vi "FVT.vi"() -> ()   [LabVIEW 2024]
uses:
  <vilib>/Utility/file.llb/Write Delimited Spreadsheet (string).vi
panel:
  in  "CompRun":bool
  out "Channel(s) (out)":u16(ring) items=["1+2", "1", "2", "3"]
  in  "Single Func Test":bool=TRUE
  in  "Position":i32 min=0 max=64 step=32
  in  "Number of Cycles":i32
  in  "Warmup Data":string[](array[string])
  out "Nominal Frequency":string="XXXXX-XXX"
  in  "Warmup":bool=TRUE
  out "Soak Time":u16(ring) items=["10", "5", "15", "30", "60", "90", "120"]
  out "Starting Time":string
  in  "Slew Time":dbl=2.0 format="%#_13g"
  out "Time Left (Estimate)":string
  out "Time":dbl
  out "PDF Path":string
  out "Time Start":timestamp
  in  "Halt Run":bool=TRUE
  out "Gatetime":string
  out "Delay Time":dbl
  out "Work Order":string
  out "Unit_Number":string
  out "System":string
  out "Path":string
  out "Frequency Address":i16=8
  out "HP Switcher Address":i32=3
  out "Oven Address":i32
  out "Temperature Array":dbl[](array[numeric])
  out "Temp Type":i32 min=1 max=15 step=1
  in  "Serial Numbers":string[](array[string])
  out "All Data":string[][][](array[string])
  in  "System Status":string
  out "Chamber":cluster{"GPIB #":u8, "Address":u8}={"GPIB #"=0, "Address"=28}
  in  "Exit":bool=TRUE
  out "Functional Test Data":string
  in  "Number of Units":i32 min=0 max=64 step=32
  in  "Functional Test":bool=TRUE
  in  "Start run":bool=TRUE
  # "FVT Test Chamber 3"
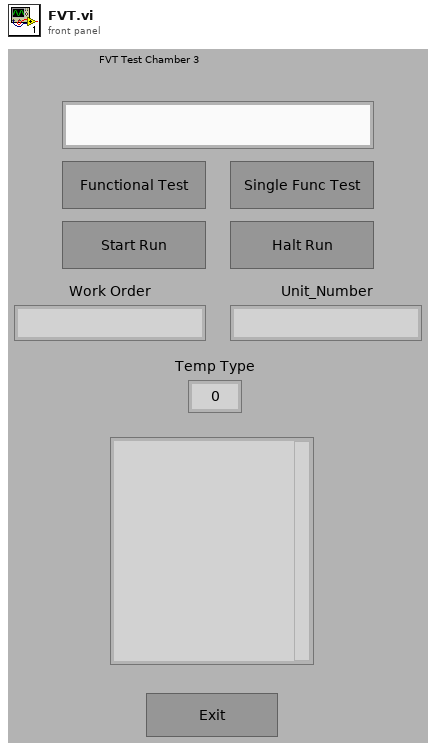
[diagram p1: front panel]
types:
  T1 = cluster{"GPIB Bus":i32, "HP Switcher Address":i32}
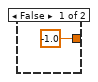
[diagram p4: hidden frame]
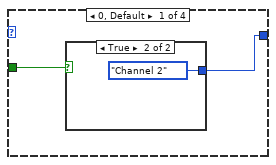
[diagram p6: hidden frame]
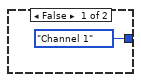
[diagram p7: hidden frame]
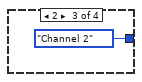
[diagram p8: hidden frame]
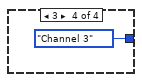
[diagram p9: hidden frame]
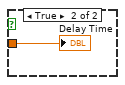
[diagram p13: hidden frame]
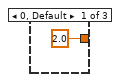
[diagram p14: hidden frame]
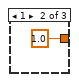
[diagram p15: hidden frame]
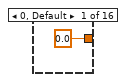
[diagram p17: hidden frame]
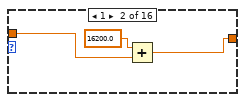
[diagram p18: hidden frame]
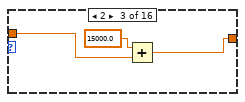
[diagram p19: hidden frame]
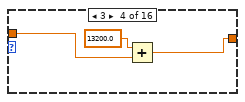
[diagram p20: hidden frame]
diagram:
  w1 = FALSE ("Exit")
  n1 = while {
    tunnel: [w15] -> w2
    stop <- w15 stop-if-true
    n2 = local read "CompRun"() -> (w10:bool)
    n3 = local write "Halt Run"(FALSE ("Halt Run")) -> ()
    n4 = local read "Start run"() -> (w17:bool)
    n5 = local read "Warmup"() -> (w12:bool)
    n6 = local read "Single Func Test"() -> (w11:bool)
    n7 = local read "Functional Test"() -> (w18:bool)
    n8 = local write "Time Left (Estimate)"("00:00:00" ("Time Left (Estimate)")) -> ()
    n9 = case shown="True" w10 {
      frame False {
      }
      frame True {
        n10 = flat-sequence {
          frame #0 {
            n11 = local write "CompRun"(FALSE ("CompRun")) -> ()
            n12 = local write "System Status"("Running Compensation Test" ("System Status")) -> ()
          }
          frame #1 {
          }
        }
      }
    }
    n13 = local write "System Status"("System Idle" ("System Status")) -> ()
    n14 = case shown="True" w12 {
      frame False {
      }
      frame True {
        n15 = flat-sequence {
          frame #0 {
            n16 = local write "Warmup"(FALSE ("Functional Test")) -> ()
            n17 = local write "System Status"("Running Warmup Test" ("System Status")) -> ()
          }
          frame #1 {
            n18 = local read "Frequency Address"() -> (w96:i16)
            n19 = local read "System"() -> (w97:string)
            n20 = call "Warmup.vi"("System"=w97, "Frequency Address"=w96) -> ()  [unwired: 10 in]
          }
        }
      }
    }
    n21 = case shown="True" w17 {
      frame False {
      }
      frame True {
        n22 = flat-sequence {
          frame #0 {
            n23 = Get Date/Time In Seconds() -> (seconds since 1Jan1904=w100:timestamp)
            n24 = Wait (ms)(milliseconds to wait=u32 5000) -> ()  [unwired: 1 out]
            n25 = Format Date/Time String(time format string (%c)="%c", seconds (now)=w100) -> (date/time string=→"Starting Time":string)  [unwired: 1 in]
            n26 = local write "System Status"("FVT running" ("System Status")) -> ()
          }
          frame #1 {
            n27 = flat-sequence {
              frame #0 {
                n28 = local read "HP Switcher Address"() -> (w104:i32)
                n29 = DevClear(3:w104, 4:0 ("GPIB Bus")) -> ()  [unwired: 1 in, 2 out]
              }
              frame #1 {
                n30 = local read "Oven Address"() -> (w106:i32)
                n31 = DevClear(3:w106, 4:0 ("GPIB Bus")) -> ()  [unwired: 1 in, 2 out]
              }
              frame #2 {
                n32 = local read "Frequency Address"() -> (w108:i16)
                n33 = DevClear(3:w108, 4:0 ("GPIB Bus")) -> ()  [unwired: 1 in, 2 out]
              }
            }
            n34 = local write "Start run"(FALSE ("Functional Test")) -> ()
          }
          frame #2 {
            n35 = call "Display Message to User"() -> ("Yes"=w120:bool)  [unwired: 10 in, 1 out]
            n36 = call "Prompt User for Input"("Enable"=w120) -> ("Seconds"=w118:dbl, "Minutes"=w114:dbl, "Hours"=w113:dbl)  [unwired: 14 in, 2 out]
            n37 = Multiply(x=w114, y=60.0) -> (x*y=w116:dbl)
            n38 = Multiply(x=w113, y=3600.0) -> (x*y=w115:dbl)
            n39 = Add(x=w115, y=w116) -> (x+y=w117:dbl)
            n40 = Add(x=w117, y=w118) -> (x+y=w119:dbl)
            n41 = Multiply(x=w119, y=1000.0) -> (x*y=w121:dbl)
            n42 = case shown="False" w120 {
              tunnel: w121 -> [_ w123]
              frame False {
                n43 = local write "Delay Time"(600000.0 ("Delay Time")) -> ()
              }
              frame True {
                "Delay Time" <- w123
              }
            }
          }
          frame #3 {
            n44 = call "Display Message to User"() -> ()  [unwired: 10 in, 2 out]
          }
          frame #4 {
            n45 = call "Parameter Setup.vi"() -> ("Serial Numbers"=w133:string[], "Slewtime (out)"=w127:u16, "Gatetime(out)"=w128:string, "Number of Units(out)"=w132:i32, "Soak Time(out)"=w125:u16, "Channel(s) (out)"=w124:u16, "Temp Type(out)"=w131:i32, "Unit_Number(out)"=w129:string, "Work Order(out)"=w130:string)  [unwired: 3 in]
            n46 = local write "Work Order"(w130) -> ()
            n47 = local write "Channel(s) (out)"(w124) -> ()
            n48 = local write "Number of Units"(w132) -> ()
            n49 = local write "Gatetime"(w128) -> ()
            n50 = case shown="2" w127 {
              tunnel: [2.0 ("Slew Time") 1.0 ("Slew Time") 0.5 ("Slew Time")] -> w126
              frame 0, Default {
              }
              frame 1 {
              }
              frame 2 {
              }
            }
            n51 = local write "Serial Numbers"(w133) -> ()
            n52 = local write "Soak Time"(w125) -> ()
            n53 = local write "Temp Type"(w131) -> ()
            n54 = local write "Unit_Number"(w129) -> ()
            n55 = local write "Slew Time"(w126) -> ()
          }
          frame #5 {
            n56 = Wait (ms)(milliseconds to wait=u32 500) -> ()  [unwired: 1 out]
          }
          frame #6 {
            w138 = "-" ("string")
            n57 = Get Date/Time In Seconds() -> (seconds since 1Jan1904=w149:timestamp)
            n58 = Format Date/Time String(time format string (%c)="%x_%I-%M" ("string"), seconds (now)=w149) -> (date/time string=w150:string)  [unwired: 1 in]
            n59 = local read "Unit_Number"() -> (w153:string)
            n60 = local read "Work Order"() -> (w152:string)
            n61 = Search and Replace String(replace all?=TRUE ("replace all? (F)"), input string=w150, search string="/", replace string="-" ("replace string (\"\")")) -> (result string=w151:string)  [unwired: 4 in, 3 out]
            n62 = Concatenate Strings("\\\\Bti-dc1\\ATE-Archive\\NewDataArchive\\_FvT\\" ("string"), "FVT-" ("string"), w152, w138, w153, w138, w151) -> (w145:string)
            n63 = local write "Path"(w145) -> ()
            n64 = String To Path(string=w145) -> (path=w146:path)
            n65 = call <vilib>:"Check if File or Folder Exists.vi"("path"=w146) -> ("file or folder exists?"=w147:bool, "dup path"=w148:path)  [unwired: 8 in, 1 out]
            n66 = case shown="False" w147 {
              tunnel: w148 -> [w154 _]
              frame False {
                n67 = Create Folder(path (use dialog)=w154) -> ()  [unwired: 2 in, 3 out]
              }
              frame True {
              }
            }
          }
          frame #7 {
            n68 = Wait (ms)(milliseconds to wait=u32 1000) -> ()  [unwired: 1 out]
          }
          frame #8 {
            n69 = flat-sequence {
              tunnel: [w161] -> w157
              tunnel: [w220] -> w156
              tunnel: w157 -> [w210]
              tunnel: w156 -> [w228]
              frame #0 {
                n70 = Get Date/Time In Seconds() -> (seconds since 1Jan1904=w162:timestamp)
                n71 = local read "Delay Time"() -> (w160:dbl)
                n72 = local write "Time Start"(w162) -> ()
                n73 = Divide(x=w160, y=1000.0) -> (x/y=w158:dbl)
                n74 = local read "Temp Type"() -> (w161:i32)
                n75 = case shown="15" w161 {
                  tunnel: w158 -> [_ w167 w170 w172 w176 w179 w182 w185 w188 w191 w194 w197 w200 w203 w206 w209]
                  tunnel: [0.0 ("Delay Time") w166 w169 w173 w175 w178 w181 w184 w187 w189 w192 w195 w198 w201 w204 w207] -> w163
                  frame 0, Default {
                  }
                  frame 1 {
                    n76 = Add(x=16200.0 ("Delay Time"), y=w167) -> (x+y=w166:dbl)
                  }
                  frame 2 {
                    n77 = Add(x=15000.0 ("Delay Time"), y=w170) -> (x+y=w169:dbl)
                  }
                  frame 3 {
                    n78 = Add(x=13200.0 ("Delay Time"), y=w172) -> (x+y=w173:dbl)
                  }
                  frame 4 {
                    n79 = Add(x=16200.0 ("Delay Time"), y=w176) -> (x+y=w175:dbl)
                  }
                  frame 5 {
                    n80 = Add(x=15000.0 ("Delay Time"), y=w179) -> (x+y=w178:dbl)
                  }
                  frame 6 {
                    n81 = Add(x=13200.0 ("Delay Time"), y=w182) -> (x+y=w181:dbl)
                  }
                  frame 7 {
                    n82 = Add(x=8400.0, y=w185) -> (x+y=w184:dbl)
                  }
                  frame 8 {
                    n83 = Add(x=14400.0 ("Delay Time"), y=w188) -> (x+y=w187:dbl)
                  }
                  frame 9 {
                    n84 = Add(x=16200.0 ("Delay Time"), y=w191) -> (x+y=w189:dbl)
                  }
                  frame 10 {
                    n85 = Add(x=15000.0 ("Delay Time"), y=w194) -> (x+y=w192:dbl)
                  }
                  frame 11 {
                    n86 = Add(x=15000.0 ("Delay Time"), y=w197) -> (x+y=w195:dbl)
                  }
                  frame 12 {
                    n87 = Add(x=15000.0 ("Delay Time"), y=w200) -> (x+y=w198:dbl)
                  }
                  frame 13 {
                    n88 = Add(x=15000.0 ("Delay Time"), y=w203) -> (x+y=w201:dbl)
                  }
                  frame 14 {
                    n89 = Add(x=15000.0 ("Delay Time"), y=w206) -> (x+y=w204:dbl)
                  }
                  frame 15 {
                    n90 = Add(x=15000.0 ("Delay Time"), y=w209) -> (x+y=w207:dbl)
                  }
                }
                "Time" <- w163
              }
              frame #1 {
                n91 = Number To Decimal String(number=w210) -> (decimal integer string=w219:string)  [unwired: 1 in]
                n92 = Concatenate Strings("\\\\BTI-dc1\\ATE\\Temp Tables\\" ("search string/char (-)"), w219, ".txt" ("string")) -> (w216:string)
                n93 = String To Path(string=w216) -> (path=w215:path)
                n94 = Read from Text File(file (use dialog)=w215, count=-1) -> (text=w214:string)  [unwired: 2 in, 3 out]
                n95 = while {
                  tunnel: [w225] -> w212 mode=indexing
                  shift-right: [w224] -> _
                  shift-left: w214 -> [w223]
                  stop <- w226 stop-if-true
                  n96 = Match Pattern(string=w223, regular expression="," ("search string/char (-)")) -> (before substring=w225:string, after substring=w224:string, offset past match=w221:i32)  [unwired: 1 in, 1 out]
                  n97 = Equal?(x=w221, y=-1) -> (x = y?=w226:bool)
                }
                n98 = Fract/Exp String To Number(string=w212) -> (number=w211:dbl[])  [unwired: 3 in, 1 out]
                "Temperature Array" <- w211
                n99 = Array Size(array=w211) -> (size(s)=w220:i32)
              }
              frame #2 {
                n100 = for {
                  N: w228 -> [_]
                  i -> [w230]
                  stop <- w229 stop-if-true
                  n101 = flat-sequence {
                    tunnel: w230 -> [w232]
                    tunnel: w230 -> [w485]
                    tunnel: w230 -> [w486]
                    frame #0 {
                      n102 = local read "Temperature Array"() -> (w238:dbl[])
                      n103 = Equal?(x=w232, y=0) -> (x = y?=w231:bool)
                      n104 = Index Array(array=w238, index=w232) -> (element=w234:dbl)
                      n105 = Number To Fractional String(number=w234) -> (F-format string=w236:string)  [unwired: 3 in]
                      n106 = case shown="False" w231 {
                        tunnel: w234 -> [w241 w333]
                        frame True {
                          n107 = flat-sequence {
                            tunnel: w241 -> [w255]
                            tunnel: [w255] -> w246
                            tunnel: [w273] -> w245
                            tunnel: [w272] -> w244
                            tunnel: w246 -> [w273]
                            tunnel: w245 -> [w279]
                            tunnel: [w279] -> w243
                            tunnel: w244 -> [w278]
                            tunnel: [w275] -> w239
                            tunnel: [w286] -> w242
                            tunnel: w243 -> [w286]
                            tunnel: [w285] -> w240
                            tunnel: w239 -> [w285]
                            tunnel: w242 -> [w289]
                            tunnel: w240 -> [w288]
                            frame #0 {
                              n108 = local read "Time Start"() -> (w253:timestamp)
                              n109 = Get Date/Time In Seconds() -> (seconds since 1Jan1904=w254:timestamp)
                              n110 = Subtract(x=w254, y=w253) -> (x-y=w251:dbl)
                              n111 = local read "Time"() -> (w250:dbl)
                              n112 = Subtract(x=w250, y=w251) -> (x-y=w248:dbl)
                              n113 = Less?(x=w248, y=0.0) -> (x < y?=w247:bool)
                              n114 = case shown="False" w247 {
                                tunnel: [w267 "00:00:00" ("time string")] -> w249
                                tunnel: w248 -> [w270 _]
                                frame False {
                                w268 = ":" ("string")
                                n115 = Quotient & Remainder(x=w270, y=3600.0) -> (x-y*floor(x/y)=w264:dbl, floor(x/y)=w266:dbl)
                                n116 = Quotient & Remainder(x=w264, y=60.0) -> (x-y*floor(x/y)=w260:dbl, floor(x/y)=w262:dbl)
                                n117 = Number To Fractional String(number=w260, precision (6)=i16 0) -> (F-format string=w259:string)  [unwired: 2 in]
                                n118 = Number To Fractional String(number=w262, precision (6)=i16 0) -> (F-format string=w261:string)  [unwired: 2 in]
                                n119 = Number To Fractional String(number=w266, precision (6)=i16 0) -> (F-format string=w265:string)  [unwired: 2 in]
                                n120 = Concatenate Strings(w265, w268, w261, w268, w259) -> (w267:string)
                                }
                                frame True {
                                }
                              }
                              n121 = local write "Time Left (Estimate)"(w249) -> ()
                            }
                            frame #1 {
                              n122 = Number To Decimal String(number=w273) -> (decimal integer string=w272:string)  [unwired: 1 in]
                            }
                            frame #2 {
                              n123 = local read "Oven Address"() -> (w274:i32)
                              n124 = Bundle(0, "Oven Address"=w274) -> (w276:cluster{i32, "Oven Address":i32})  [unwired: 1 in]
                              n125 = while {
                                tunnel: w278 -> [w284]
                                tunnel: w276 -> [w281]
                                tunnel: [w281] -> w275
                                stop <- w282 continue-if-true
                                n126 = call "Set Temperature and Rise Time2023.vi"("Slew Time String"="0", "Temperature String"=w284, "Device"=w281) -> ("error out"=w283:errorcluster)  [unwired: 3 in]
                                n127 = Unbundle By Name(w283) -> ("status"=w282:bool)
                              }
                            }
                            frame #3 {
                              n128 = Wait (ms)(milliseconds to wait=u32 1000) -> ()  [unwired: 1 out]
                            }
                            frame #4 {
                              n129 = while {
                                tunnel: w289 -> [w293]
                                tunnel: w288 -> [w290]
                                stop <- w291 stop-if-true
                                n130 = flat-sequence {
                                tunnel: w293 -> [w303]
                                tunnel: [w295] -> w292
                                tunnel: w290 -> [w294]
                                tunnel: w292 -> [w332]
                                tunnel: [w331] -> w291
                                frame #0 {
                                n131 = call "Read Saunders Temperature2023.vi"("Device"=w294) -> ("error out 2"=w296:errorcluster, "Temperature"=w298:dbl)  [unwired: 3 in]
                                n132 = Add(x=0.5, y=w303) -> (x+y=w299:dbl)
                                n133 = Subtract(x=w303, y=0.5) -> (x-y=w301:dbl)
                                n134 = Unbundle By Name(w296) -> ("status"=w297:bool)
                                n135 = In Range and Coerce(upper limit=w299, x=w298, lower limit=w301) -> (In Range?=w295:bool)  [unwired: 1 out]
                                n136 = case shown="False" w297 {
                                frame False {
                                }
                                frame True {
                                n137 = local read "Oven Address"() -> (w304:i32)
                                n138 = DevClear(3:w304, 4:0 ("GPIB Bus")) -> ()  [unwired: 1 in, 2 out]
                                }
                                }
                                }
                                frame #1 {
                                n139 = local read "Time Start"() -> (w312:timestamp)
                                n140 = Get Date/Time In Seconds() -> (seconds since 1Jan1904=w313:timestamp)
                                n141 = Subtract(x=w313, y=w312) -> (x-y=w310:dbl)
                                n142 = local read "Time"() -> (w311:dbl)
                                n143 = Subtract(x=w311, y=w310) -> (x-y=w307:dbl)
                                n144 = Less?(x=w307, y=0.0) -> (x < y?=w308:bool)
                                n145 = case shown="False" w308 {
                                tunnel: [w325 "00:00:00" ("time string")] -> w306
                                tunnel: w307 -> [w328 _]
                                frame False {
                                w326 = ":" ("string")
                                n146 = Quotient & Remainder(x=w328, y=3600.0) -> (x-y*floor(x/y)=w322:dbl, floor(x/y)=w324:dbl)
                                n147 = Quotient & Remainder(x=w322, y=60.0) -> (x-y*floor(x/y)=w318:dbl, floor(x/y)=w320:dbl)
                                n148 = Number To Fractional String(number=w318, precision (6)=i16 0) -> (F-format string=w317:string)  [unwired: 2 in]
                                n149 = Number To Fractional String(number=w320, precision (6)=i16 0) -> (F-format string=w319:string)  [unwired: 2 in]
                                n150 = Number To Fractional String(number=w324, precision (6)=i16 0) -> (F-format string=w323:string)  [unwired: 2 in]
                                n151 = Concatenate Strings(w323, w326, w319, w326, w317) -> (w325:string)
                                }
                                frame True {
                                }
                                }
                                n152 = local write "Time Left (Estimate)"(w306) -> ()
                                }
                                frame #2 {
                                n153 = local read "Halt Run"() -> (w330:bool)
                                n154 = Or(x=w330, y=w332) -> (x .or. y?=w331:bool)
                                }
                                }
                              }
                            }
                          }
                        }
                        frame False {
                          n155 = flat-sequence {
                            tunnel: w333 -> [w358]
                            tunnel: [w358] -> w349
                            tunnel: [w382] -> w348
                            tunnel: [w381] -> w347
                            tunnel: [w376] -> w346
                            tunnel: [w380] -> w345
                            tunnel: w349 -> [w382]
                            tunnel: w348 -> [w402]
                            tunnel: [w402] -> w344
                            tunnel: [w403] -> w343
                            tunnel: w347 -> [w405]
                            tunnel: [w405] -> w342
                            tunnel: w346 -> [w404]
                            tunnel: w345 -> [w401]
                            tunnel: [w426] -> w341
                            tunnel: w344 -> [w425]
                            tunnel: w343 -> [w424]
                            tunnel: w342 -> [w426]
                            tunnel: [w425] -> w340
                            tunnel: [w424] -> w339
                            tunnel: [w423] -> w338
                            tunnel: w341 -> [w427]
                            tunnel: [w427] -> w337
                            tunnel: w340 -> [w430]
                            tunnel: [w430] -> w336
                            tunnel: w339 -> [w429]
                            tunnel: w338 -> [w428]
                            tunnel: [w437] -> w335
                            tunnel: w337 -> [w437]
                            tunnel: [w436] -> w334
                            tunnel: w336 -> [w436]
                            tunnel: w335 -> [w440]
                            tunnel: w334 -> [w439]
                            frame #0 {
                              n156 = local read "Time Start"() -> (w356:timestamp)
                              n157 = Get Date/Time In Seconds() -> (seconds since 1Jan1904=w357:timestamp)
                              n158 = Subtract(x=w357, y=w356) -> (x-y=w353:dbl)
                              n159 = local read "Time"() -> (w354:dbl)
                              n160 = Subtract(x=w354, y=w353) -> (x-y=w350:dbl)
                              n161 = Less?(x=w350, y=0.0) -> (x < y?=w351:bool)
                              n162 = case shown="False" w351 {
                                tunnel: [w370 "00:00:00" ("time string")] -> w352
                                tunnel: w350 -> [w373 _]
                                frame False {
                                w371 = ":" ("string")
                                n163 = Quotient & Remainder(x=w373, y=3600.0) -> (x-y*floor(x/y)=w367:dbl, floor(x/y)=w369:dbl)
                                n164 = Quotient & Remainder(x=w367, y=60.0) -> (x-y*floor(x/y)=w363:dbl, floor(x/y)=w365:dbl)
                                n165 = Number To Fractional String(number=w363, precision (6)=i16 0) -> (F-format string=w362:string)  [unwired: 2 in]
                                n166 = Number To Fractional String(number=w365, precision (6)=i16 0) -> (F-format string=w364:string)  [unwired: 2 in]
                                n167 = Number To Fractional String(number=w369, precision (6)=i16 0) -> (F-format string=w368:string)  [unwired: 2 in]
                                n168 = Concatenate Strings(w368, w371, w364, w371, w362) -> (w370:string)
                                }
                                frame True {
                                }
                              }
                              n169 = local write "Time Left (Estimate)"(w352) -> ()
                            }
                            frame #1 {
                              n170 = local read "Oven Address"() -> (w375:i32)
                              n171 = Bundle(0, "Oven Address"=w375) -> (w381:cluster{i32, "Oven Address":i32})  [unwired: 1 in]
                              n172 = call "Read Saunders Temperature2023.vi"("Device"=w381) -> ("error out 2"=w378:errorcluster, "Temperature"=w377:dbl)  [unwired: 3 in]
                              n173 = Unbundle By Name(w378) -> ("status"=w379:bool)
                              n174 = case shown="False" w379 {
                                tunnel: w377 -> [w394 w399]
                                tunnel: [w394 w396] -> w376
                                frame False {
                                }
                                frame True {
                                n175 = In Range and Coerce(upper limit=100.0, x=w399, lower limit=-50.0) -> (coerced(x)=w396:dbl)  [unwired: 1 out]
                                n176 = local read "Oven Address"() -> (w395:i32)
                                n177 = DevClear(3:w395, 4:0 ("GPIB Bus")) -> ()  [unwired: 1 in, 2 out]
                                }
                              }
                              n178 = Greater?(x=w382, y=0) -> (0:w390:bool)
                              n179 = Less?(x=w382, y=0.0) -> (x < y?=w387:bool)
                              n180 = Less?(x=w376, y=0.0) -> (x < y?=w389:bool)
                              n181 = Greater?(x=w376, y=0.0) -> (0:w388:bool)
                              n182 = And(x=w390, y=w389) -> (x .and. y?=w386:bool)
                              n183 = And(x=w388, y=w387) -> (x .and. y?=w383:bool)
                              n184 = Or(x=w386, y=w383) -> (x .or. y?=w380:bool)
                            }
                            frame #2 {
                              n185 = case shown="True" w401 {
                                tunnel: w404 -> [w411 w419]
                                tunnel: w402 -> [w412 w420]
                                tunnel: [w408 w416] -> w403
                                frame False {
                                n186 = Subtract(x=w412, y=w411) -> (x-y=w410:dbl)
                                n187 = local read "Slew Time"() -> (w406:dbl)
                                n188 = Absolute Value(x=w410) -> (abs(x)=w407:dbl)
                                n189 = Quotient & Remainder(x=w407, y=w406) -> (floor(x/y)=w409:dbl)  [unwired: 1 out]
                                n190 = Number To Decimal String(number=w409) -> (decimal integer string=w408:string)  [unwired: 1 in]
                                }
                                frame True {
                                n191 = Absolute Value(x=w420) -> (abs(x)=w417:dbl)
                                n192 = Absolute Value(x=w419) -> (abs(x)=w418:dbl)
                                n193 = local read "Slew Time"() -> (w413:dbl)
                                n194 = Add(x=w417, y=w418) -> (x+y=w414:dbl)
                                n195 = Quotient & Remainder(x=w414, y=w413) -> (floor(x/y)=w415:dbl)  [unwired: 1 out]
                                n196 = Number To Decimal String(number=w415) -> (decimal integer string=w416:string)  [unwired: 1 in]
                                }
                              }
                            }
                            frame #3 {
                              n197 = local read "Oven Address"() -> (w421:i32)
                              n198 = Number To Decimal String(number=w425) -> (decimal integer string=w423:string)  [unwired: 1 in]
                              n199 = DevClear(3:w421, 4:0 ("GPIB Bus")) -> ()  [unwired: 1 in, 2 out]
                            }
                            frame #4 {
                              n200 = while {
                                tunnel: w429 -> [w435]
                                tunnel: w428 -> [w434]
                                tunnel: w427 -> [w433]
                                stop <- w431 continue-if-true
                                n201 = call "Set Temperature and Rise Time2023.vi"("Slew Time String"=w435, "Temperature String"=w434, "Device"=w433) -> ("error out"=w432:errorcluster)  [unwired: 3 in]
                                n202 = Unbundle By Name(w432) -> ("status"=w431:bool)
                              }
                            }
                            frame #5 {
                              n203 = Wait (ms)(milliseconds to wait=u32 1000) -> ()  [unwired: 1 out]
                            }
                            frame #6 {
                              n204 = while {
                                tunnel: w440 -> [w443]
                                tunnel: w439 -> [w444]
                                stop <- w441 stop-if-true
                                n205 = flat-sequence {
                                tunnel: w444 -> [w454]
                                tunnel: w443 -> [w449]
                                tunnel: [w445] -> w442
                                tunnel: w442 -> [w483]
                                tunnel: [w482] -> w441
                                frame #0 {
                                n206 = call "Read Saunders Temperature2023.vi"("Device"=w449) -> ("error out 2"=w446:errorcluster, "Temperature"=w448:dbl)  [unwired: 3 in]
                                n207 = Add(x=0.5, y=w454) -> (x+y=w450:dbl)
                                n208 = Subtract(x=w454, y=0.5) -> (x-y=w452:dbl)
                                n209 = Unbundle By Name(w446) -> ("status"=w447:bool)
                                n210 = In Range and Coerce(upper limit=w450, x=w448, lower limit=w452) -> (In Range?=w445:bool)  [unwired: 1 out]
                                n211 = case shown="False" w447 {
                                frame False {
                                }
                                frame True {
                                n212 = local read "Oven Address"() -> (w455:i32)
                                n213 = DevClear(3:w455, 4:0 ("GPIB Bus")) -> ()  [unwired: 1 in, 2 out]
                                }
                                }
                                }
                                frame #1 {
                                n214 = local read "Time Start"() -> (w463:timestamp)
                                n215 = Get Date/Time In Seconds() -> (seconds since 1Jan1904=w464:timestamp)
                                n216 = Subtract(x=w464, y=w463) -> (x-y=w460:dbl)
                                n217 = local read "Time"() -> (w461:dbl)
                                n218 = Subtract(x=w461, y=w460) -> (x-y=w457:dbl)
                                n219 = Less?(x=w457, y=0.0) -> (x < y?=w458:bool)
                                n220 = case shown="False" w458 {
                                tunnel: [w476 "00:00:00" ("time string")] -> w459
                                tunnel: w457 -> [w479 _]
                                frame False {
                                w477 = ":" ("string")
                                n221 = Quotient & Remainder(x=w479, y=3600.0) -> (x-y*floor(x/y)=w473:dbl, floor(x/y)=w475:dbl)
                                n222 = Quotient & Remainder(x=w473, y=60.0) -> (x-y*floor(x/y)=w469:dbl, floor(x/y)=w471:dbl)
                                n223 = Number To Fractional String(number=w469, precision (6)=i16 0) -> (F-format string=w468:string)  [unwired: 2 in]
                                n224 = Number To Fractional String(number=w471, precision (6)=i16 0) -> (F-format string=w470:string)  [unwired: 2 in]
                                n225 = Number To Fractional String(number=w475, precision (6)=i16 0) -> (F-format string=w474:string)  [unwired: 2 in]
                                n226 = Concatenate Strings(w474, w477, w470, w477, w468) -> (w476:string)
                                }
                                frame True {
                                }
                                }
                                n227 = local write "Time Left (Estimate)"(w459) -> ()
                                }
                                frame #2 {
                                n228 = local read "Halt Run"() -> (w481:bool)
                                n229 = Or(x=w481, y=w483) -> (x .or. y?=w482:bool)
                                }
                                }
                              }
                            }
                          }
                        }
                      }
                      n230 = Concatenate Strings("Setting Temperature to " ("System Status"), w236) -> (w235:string)
                      n231 = local write "System Status"(w235) -> ()
                    }
                    frame #1 {
                      n232 = local read "Halt Run"() -> (w484:bool)
                      n233 = case shown="False" w484 {
                        tunnel: w486 -> [w488 _]
                        tunnel: w485 -> [w487 _]
                        frame False {
                          n234 = flat-sequence {
                            tunnel: w488 -> [w490]
                            tunnel: w487 -> [w504]
                            frame #0 {
                              n235 = Equal?(x=w490, y=0) -> (x = y?=w489:bool)
                              n236 = case shown="True" w489 {
                                frame False {
                                }
                                frame True {
                                n237 = local read "Delay Time"() -> (w492:dbl)
                                n238 = Wait (ms)(milliseconds to wait=w492) -> ()  [unwired: 1 out]
                                }
                              }
                            }
                            frame #1 {
                              n239 = local read "Soak Time"() -> (w495:u16)
                              n240 = local read "HP Switcher Address"() -> (w494:i32)
                              n241 = case shown="2" w495 {
                                frame 0, Default {
                                n242 = Wait (ms)(milliseconds to wait=u32 600000) -> ()  [unwired: 1 out]
                                }
                                frame 1 {
                                n243 = Wait (ms)(milliseconds to wait=u32 300000) -> ()  [unwired: 1 out]
                                }
                                frame 2 {
                                n244 = Wait (ms)(milliseconds to wait=u32 10) -> ()  [unwired: 1 out]
                                }
                                frame 3 {
                                n245 = Wait (ms)(milliseconds to wait=u32 900000) -> ()  [unwired: 1 out]
                                }
                                frame 4 {
                                n246 = Wait (ms)(milliseconds to wait=u32 1800000) -> ()  [unwired: 1 out]
                                }
                                frame 5 {
                                n247 = Wait (ms)(milliseconds to wait=u32 3600000) -> ()  [unwired: 1 out]
                                }
                                frame 6 {
                                n248 = Wait (ms)(milliseconds to wait=u32 5400000) -> ()  [unwired: 1 out]
                                }
                                frame 7 {
                                n249 = Wait (ms)(milliseconds to wait=u32 7200000) -> ()  [unwired: 1 out]
                                }
                              }
                              n250 = call "HP3488A Reset(GPIB).vi"("Address"=w494, "GPIB#"=0 ("GPIB Bus")) -> ()  [unwired: 3 in, 1 out]
                            }
                            frame #2 {
                              n251 = local read "Number of Units"() -> (w506:i32)
                              n252 = local read "Serial Numbers"() -> (w505:string[])
                              n253 = for {
                                N: w506 -> [_]
                                tunnel: w505 -> [w513] mode=indexing
                                tunnel: w504 -> [w517]
                                i -> [w522]
                                stop <- w512 stop-if-true
                                n254 = Increment(x=w522) -> (x+1=w514:i32)
                                n255 = flat-sequence {
                                tunnel: w514 -> [w527]
                                tunnel: [w527] -> w511
                                tunnel: [w536] -> w510
                                tunnel: w511 -> [w536]
                                tunnel: w510 -> [w554]
                                tunnel: [w554] -> w509
                                tunnel: [w561] -> w521
                                tunnel: [w560] -> w520
                                tunnel: w509 -> [w561]
                                tunnel: [w566] -> w519
                                tunnel: w521 -> [w565]
                                tunnel: w519 -> [w628]
                                tunnel: [w628] -> w518
                                tunnel: w517 -> [w627]
                                tunnel: [w621] -> w516
                                tunnel: [w620] -> w515
                                tunnel: w514 -> [w622]
                                tunnel: w513 -> [w619]
                                tunnel: w518 -> [w652]
                                tunnel: w520 -> [w671]
                                tunnel: w513 -> [w656]
                                tunnel: w516 -> [w654]
                                tunnel: w515 -> [w664]
                                tunnel: [w658] -> w507
                                tunnel: [w672] -> w508
                                tunnel: w507 -> [w672]
                                tunnel: w508 -> [w674]
                                frame #0 {
                                n256 = Wait (ms)(milliseconds to wait=u32 1000) -> ()  [unwired: 1 out]
                                n257 = Number To Decimal String(number=w527) -> (decimal integer string=w524:string)  [unwired: 1 in]
                                n258 = Concatenate Strings("Reading for Position " ("System Status"), w524) -> (w523:string)
                                n259 = local write "System Status"(w523) -> ()
                                }
                                frame #1 {
                                n260 = local read "Time Start"() -> (w531:timestamp)
                                n261 = Get Date/Time In Seconds() -> (seconds since 1Jan1904=w535:timestamp)
                                n262 = Subtract(x=w535, y=w531) -> (x-y=w530:dbl)
                                n263 = local read "Time"() -> (w529:dbl)
                                n264 = Subtract(x=w529, y=w530) -> (x-y=w534:dbl)
                                n265 = Less?(x=w534, y=0.0) -> (x < y?=w532:bool)
                                n266 = case shown="False" w532 {
                                tunnel: [w548 "00:00:00" ("time string")] -> w528
                                tunnel: w534 -> [w551 _]
                                frame False {
                                w549 = ":" ("string")
                                n267 = Quotient & Remainder(x=w551, y=3600.0) -> (x-y*floor(x/y)=w545:dbl, floor(x/y)=w547:dbl)
                                n268 = Quotient & Remainder(x=w545, y=60.0) -> (x-y*floor(x/y)=w541:dbl, floor(x/y)=w543:dbl)
                                n269 = Number To Fractional String(number=w541, precision (6)=i16 0) -> (F-format string=w540:string)  [unwired: 2 in]
                                n270 = Number To Fractional String(number=w543, precision (6)=i16 0) -> (F-format string=w542:string)  [unwired: 2 in]
                                n271 = Number To Fractional String(number=w547, precision (6)=i16 0) -> (F-format string=w546:string)  [unwired: 2 in]
                                n272 = Concatenate Strings(w546, w549, w542, w549, w540) -> (w548:string)
                                }
                                frame True {
                                }
                                }
                                n273 = local write "Time Left (Estimate)"(w528) -> ()
                                }
                                frame #2 {
                                n274 = Wait (ms)(milliseconds to wait=u32 1000) -> ()  [unwired: 1 out]
                                }
                                frame #3 {
                                n275 = local read "Oven Address"() -> (w555:i32)
                                n276 = Bundle(0, "Oven Address"=w555) -> (w557:cluster{i32, "Oven Address":i32})  [unwired: 1 in]
                                n277 = call "Read Saunders Temperature2023.vi"("Device"=w557) -> ("error out 2"=w558:errorcluster, "Temperature"=w560:dbl)  [unwired: 3 in]
                                n278 = Unbundle By Name(w558) -> ("status"=w559:bool)
                                n279 = case shown="False" w559 {
                                frame False {
                                }
                                frame True {
                                n280 = local read "Oven Address"() -> (w562:i32)
                                n281 = DevClear(3:w562, 4:0 ("GPIB Bus")) -> ()  [unwired: 1 in, 2 out]
                                }
                                }
                                }
                                frame #4 {
                                n282 = for {
                                N: 10 -> [_]
                                tunnel: [w574] -> w566
                                tunnel: w565 -> [w573]
                                stop <- w568 stop-if-true
                                n283 = flat-sequence {
                                tunnel: w573 -> [w578]
                                tunnel: [w578] -> w576
                                tunnel: [w577] -> w572
                                tunnel: w576 -> [w589]
                                tunnel: [w589] -> w575
                                tunnel: [w608] -> w570
                                tunnel: [w609] -> w574
                                tunnel: w575 -> [w592]
                                frame #0 {
                                n284 = local read "HP Switcher Address"() -> (w582:i32)
                                n285 = Bundle(0, "HP Switcher Address"=w582) -> (w580:cluster{i32, "HP Switcher Address":i32})  [unwired: 1 in]
                                n286 = call "Close HP3488A Switcher(GPIB).vi"("Device In"=w580, "reset"=FALSE, "Use Card# 5"=TRUE, "ID query"=FALSE, "error in (no error)"=errorcluster {"status"=FALSE, "code"=0, "source"=""}, "Position Number"=w578) -> ("error out"=w579:errorcluster)  [unwired: 2 in]
                                n287 = Unbundle By Name(w579) -> ("status"=w577:bool)
                                n288 = case shown="True" w577 {
                                frame False {
                                }
                                frame True {
                                n289 = local read "HP Switcher Address"() -> (w587:i32)
                                n290 = call "HP3488A Reset(GPIB).vi"("Address"=w587, "GPIB#"=0 ("GPIB Bus")) -> ()  [unwired: 3 in, 1 out]
                                }
                                }
                                }
                                frame #1 {
                                n291 = Wait (ms)(milliseconds to wait=u32 1000) -> ()  [unwired: 1 out]
                                }
                                frame #2 {
                                n292 = local read "Channel(s) (out)"() -> (w595:u16)
                                n293 = Greater?(x=w592, y=16) -> (0:w591:bool)
                                n294 = case shown="3" w595 {
                                tunnel: [w611 enum16{"Channel 1", "Channel 2", "Channel 3"}."Channel 1" ("Channel(1,2,3)") enum16{"Channel 1", "Channel 2", "Channel 3"}."Channel 2" ("Channel(1,2,3)") enum16{"Channel 1", "Channel 2", "Channel 3"}."Channel 3" ("Channel(1,2,3)")] -> w594
                                tunnel: w591 -> [w610 _ _ _]
                                frame 0, Default {
                                n295 = case shown="True" w610 {
                                tunnel: [enum16{"Channel 1", "Channel 2", "Channel 3"}."Channel 1" ("Channel(1,2,3)") enum16{"Channel 1", "Channel 2", "Channel 3"}."Channel 2" ("Channel(1,2,3)")] -> w611
                                frame False {
                                }
                                frame True {
                                }
                                }
                                }
                                frame 1 {
                                }
                                frame 2 {
                                }
                                frame 3 {
                                }
                                }
                                n296 = local read "Gatetime"() -> (w606:string)
                                n297 = local read "Frequency Address"() -> (w605:i16)
                                n298 = Fract/Exp String To Number(string=w606) -> (number=w607:dbl)  [unwired: 3 in, 1 out]
                                n299 = call "HP53131 Measure Frequency2023.vi"("GPIB Bus"=0, "Number of Readings"=1, "GPIB Address"=w605, "Gate Time"=w607, "Channel(1,2,3)"=w594) -> ("error out"=w603:errorcluster, "Frequency"=w596:dbl)  [unwired: 1 in]
                                n300 = Unbundle By Name(w603) -> ("status"=w602:bool)
                                n301 = In Range and Coerce(upper limit=5000000000.0, x=w596, lower limit=0.0) -> (coerced(x)=w604:dbl)  [unwired: 1 out]
                                n302 = case shown="False" w602 {
                                frame False {
                                }
                                frame True {
                                n303 = local read "Frequency Address"() -> (w617:i16)
                                n304 = DevClear(3:w617, 4:0 ("GPIB Bus")) -> ()  [unwired: 1 in, 2 out]
                                }
                                }
                                n305 = Not Equal?(x=w596, y=0.0) -> (x != y?=w608:bool)
                                n306 = Number To Fractional String(number=w604) -> (F-format string=w609:string)  [unwired: 3 in]
                                }
                                }
                                n307 = Not(x=w572) -> (.not. x?=w571:bool)
                                n308 = local read "Halt Run"() -> (w567:bool)
                                n309 = And(x=w570, y=w571) -> (x .and. y?=w569:bool)
                                n310 = Or(x=w569, y=w567) -> (x .or. y?=w568:bool)
                                }
                                }
                                frame #5 {
                                n311 = local read "Path"() -> (w626:string)
                                n312 = Concatenate Strings(w626, "\\" ("string"), w619, ".csv" ("string")) -> (w623:string)
                                n313 = String To Path(string=w623) -> (path=w620:path)
                                n314 = case shown="0" w627 {
                                tunnel: w620 -> [w644 _]
                                frame 0 {
                                n315 = Build Array("Unit_Number" ("string"), "Serial_Number" ("element"), "Date_Code" ("element"), "Work_Order" ("element"), "Test_System" ("element"), "Position" ("element"), "Fixture_SN" ("element"), "Run_FileName" ("element"), "Frequency" ("element"), "Temperature" ("element"), "Time_stamp" ("element"), "Run_ID" ("element")) -> (w643:string[])
                                n316 = call-poly <vilib>:"Write Delimited Spreadsheet.vi"("file path (dialog if empty)"=w644, "1D data"=w643, "append to file? (new file:F)"=FALSE, "delimiter (\\t)"="," ("delimiter (\\t)")) -> ()  [unwired: 10 in, 2 out]
                                }
                                frame 1, Default {
                                }
                                }
                                n317 = Number To Decimal String(number=w622) -> (decimal integer string=w621:string)  [unwired: 1 in]
                                }
                                frame #6 {
                                w647 = "','" ("element")
                                n318 = Get Date/Time In Seconds() -> (seconds since 1Jan1904=w670:timestamp)
                                n319 = local read "Temp Type"() -> (w660:i32)
                                n320 = local read "Slew Time"() -> (w659:dbl)
                                n321 = local read "Unit_Number"() -> (w653:string)
                                n322 = local read "Starting Time"() -> (w646:string)
                                n323 = local read "Work Order"() -> (w669:string)
                                n324 = Format Date/Time String(time format string (%c)="%c", seconds (now)=w670) -> (date/time string=w648:string)  [unwired: 1 in]
                                n325 = Number To Fractional String(number=w671) -> (F-format string=w651:string)  [unwired: 3 in]
                                n326 = Number To Decimal String(number=w660) -> (decimal integer string=w650:string)  [unwired: 1 in]
                                n327 = Number To Fractional String(number=w659) -> (F-format string=w649:string)  [unwired: 3 in]
                                n328 = local read "System"() -> (w655:string)
                                n329 = Concatenate Strings("INSERT INTO FVT\nVALUES('" ("element"), w656, w647, w653, w647, w655, w647, w654, w647, w653, w647, w652, w647, w651, w647, w650, w647, w649, w647, w648, w647, w646, "')" ("Unit_Number")) -> (w658:string)
                                n330 = Build Array(w653, w656, w656, w669, w655, w654, "" ("element"), "NONE" ("element"), w652, w651, w648, "1313" ("element")) -> (w661:string[])
                                n331 = call-poly <vilib>:"Write Delimited Spreadsheet.vi"("file path (dialog if empty)"=w664, "1D data"=w661, "append to file? (new file:F)"=TRUE, "delimiter (\\t)"="," ("delimiter (\\t)")) -> ()  [unwired: 10 in, 2 out]
                                }
                                frame #7 {
                                n332 = Wait (ms)(milliseconds to wait=u32 500) -> ()  [unwired: 1 out]
                                }
                                frame #8 {
                                n333 = call "Database Sending.vi"("Command"=w674) -> ()  [unwired: 11 in]
                                }
                                }
                                n334 = local read "Halt Run"() -> (w512:bool)
                              }
                            }
                          }
                        }
                        frame True {
                        }
                      }
                    }
                  }
                  n335 = local read "Halt Run"() -> (w229:bool)
                }
              }
            }
          }
          frame #9 {
            n336 = local read "Oven Address"() -> (w676:i32)
            n337 = Bundle(0, "Oven Address"=w676) -> (w675:cluster{i32, "Oven Address":i32})  [unwired: 1 in]
            n338 = call "Set Temperature and Rise Time2023.vi"("Temperature String"="O", "Device"=w675) -> ()  [unwired: 4 in, 1 out]
          }
          frame #10 {
            n339 = local read "Halt Run"() -> (w680:bool)
            n340 = Not(x=w680) -> (.not. x?=w679:bool)
            n341 = case shown="True" w679 {
              frame False {
              }
              frame True {
                n342 = local read "Number of Units"() -> (w681:i32)
                n343 = for {
                  N: w681 -> [_]
                  i -> [w683]
                  n344 = flat-sequence {
                    tunnel: w683 -> [w696]
                    tunnel: [w694] -> w682
                    tunnel: w682 -> [w710]
                    frame #0 {
                      n345 = Wait (ms)(milliseconds to wait=u32 1000) -> ()  [unwired: 1 out]
                      n346 = local write "System Status"("Converting Files to Winplot PDFs") -> ()
                    }
                    frame #1 {
                      w687 = "-" ("string")
                      n347 = Get Date/Time In Seconds() -> (seconds since 1Jan1904=w693:timestamp)
                      n348 = Format Date/Time String(time format string (%c)="%x_%I-%M" ("string"), seconds (now)=w693) -> (date/time string=w689:string)  [unwired: 1 in]
                      n349 = local read "Serial Numbers"() -> (w697:string[])
                      n350 = local read "Unit_Number"() -> (w705:string)
                      n351 = local read "Work Order"() -> (w706:string)
                      n352 = Search and Replace String(replace all?=TRUE ("replace all? (F)"), input string=w689, search string="/", replace string="-" ("replace string (\"\")")) -> (result string=w686:string)  [unwired: 4 in, 3 out]
                      n353 = Concatenate Strings("\\\\Bti-dc1\\ate\\Winplots\\" ("string"), "FVT-" ("string"), w706, w687, w705, w687, w686) -> (w699:string)
                      n354 = Index Array(array=w697, index=w696) -> (element=w694:string)
                      n355 = String To Path(string=w699) -> (path=w702:path)
                      n356 = call <vilib>:"Check if File or Folder Exists.vi"("path"=w702) -> ("file or folder exists?"=w703:bool, "dup path"=w704:path)  [unwired: 8 in, 1 out]
                      n357 = Concatenate Strings(w699, "\\" ("string"), w694) -> (w695:string)
                      n358 = case shown="False" w703 {
                        tunnel: w704 -> [w707 _]
                        frame False {
                          n359 = Create Folder(path (use dialog)=w707) -> ()  [unwired: 2 in, 3 out]
                        }
                        frame True {
                        }
                      }
                      n360 = local write "PDF Path"(w695) -> ()
                    }
                    frame #2 {
                      n361 = local read "Path"() -> (w712:string)
                      n362 = Concatenate Strings(w712, "\\" ("string"), w710, ".csv" ("string")) -> (w708:string)
                      n363 = local read "PDF Path"() -> (w721:string)
                      n364 = Open Python Session(python version="3.12" ("Python version")) -> (session out=w720:refnum<k35>, error out=w719:errorcluster)  [unwired: 2 in]
                      n365 = node(w720, path "C:/Users/presentation/Desktop/FVT FIXER/convert.py" ("module path"), "load_data" ("function name"), w719, string[] [], w708, w721) -> (w718:refnum<k35>, w717:errorcluster)  [unwired: 3 in, 2 out]
                      n366 = Close Python Session(session in=w718, error in=w717) -> ()  [unwired: 1 out]
                    }
                  }
                }
              }
            }
          }
          frame #11 {
            n367 = invoke on="Temp Type" class="DigNum (strict)" method="Reinit To Default"() -> ()  [unwired: 3 in, 3 out]
            n368 = invoke on="Unit_Number" class="Str" method="Reinit To Default"() -> ()  [unwired: 3 in, 3 out]
            n369 = invoke on="Work Order" class="Str" method="Reinit To Default"() -> ()  [unwired: 3 in, 3 out]
            n370 = local write "Halt Run"(FALSE ("Halt Run")) -> ()
          }
        }
      }
    }
    n371 = case shown="True" w11 {
      frame False {
      }
      frame True {
        n372 = flat-sequence {
          tunnel: [w26] -> w21
          tunnel: [w30] -> w22
          tunnel: w21 -> [w28]
          tunnel: w22 -> [w92]
          frame #0 {
            n373 = local write "Single Func Test"(FALSE ("Functional Test")) -> ()
            n374 = local write "System Status"("Running Single Functional Test" ("System Status")) -> ()
          }
          frame #1 {
            n375 = call "Parameter Setup( Single Functional).vi"() -> ("Run?"=w26:bool, "Position(out)"=w27:i32, "Channel(s) (out)"=w25:u16)  [unwired: 9 in]
            n376 = local write "Channel(s) (out)"(w25) -> ()
            n377 = local write "Position"(w27) -> ()
          }
          frame #2 {
            n378 = case shown="True" w28 {
              tunnel: [-1.0 ("upper limit") w32] -> w29
              frame False {
              }
              frame True {
                n379 = flat-sequence {
                  tunnel: [w42] -> w32
                  frame #0 {
                    n380 = Wait (ms)(milliseconds to wait=u32 500) -> ()  [unwired: 1 out]
                  }
                  frame #1 {
                    n381 = flat-sequence {
                      frame #0 {
                        n382 = local read "HP Switcher Address"() -> (w34:i32)
                        n383 = DevClear(3:w34, 4:0 ("GPIB Bus")) -> ()  [unwired: 1 in, 2 out]
                      }
                      frame #1 {
                        n384 = local read "Oven Address"() -> (w36:i32)
                        n385 = DevClear(3:w36, 4:0 ("GPIB Bus")) -> ()  [unwired: 1 in, 2 out]
                      }
                      frame #2 {
                        n386 = local read "Frequency Address"() -> (w38:i16)
                        n387 = DevClear(3:w38, 4:0 ("GPIB Bus")) -> ()  [unwired: 1 in, 2 out]
                      }
                    }
                  }
                  frame #2 {
                    n388 = Wait (ms)(milliseconds to wait=u32 100) -> ()  [unwired: 1 out]
                  }
                  frame #3 {
                    n389 = for {
                      N: 10 -> [_]
                      tunnel: [w49] -> w42
                      stop <- w43 stop-if-true
                      n390 = flat-sequence {
                        tunnel: [w52] -> w51
                        tunnel: [w53] -> w46
                        tunnel: [w64] -> w50
                        tunnel: w51 -> [w64]
                        tunnel: [w74] -> w49
                        tunnel: w50 -> [w73]
                        tunnel: [w70] -> w48
                        frame #0 {
                          n391 = local read "HP Switcher Address"() -> (w59:i32)
                          n392 = local read "Position"() -> (w52:i32)
                          n393 = Bundle("GPIB Bus"=0, "HP Switcher Address"=w59) -> (w60:T1)  [unwired: 1 in]
                          n394 = call "Close HP3488A Switcher(GPIB).vi"("Device In"=w60, "reset"=FALSE, "Use Card# 5"=TRUE, "ID query"=FALSE, "error in (no error)"=errorcluster {"status"=FALSE, "code"=0, "source"=""}, "Position Number"=w52) -> ("error out"=w61:errorcluster)  [unwired: 2 in]
                          n395 = Unbundle By Name(w61) -> ("status"=w53:bool)
                          n396 = case shown="True" w53 {
                            frame False {
                            }
                            frame True {
                              n397 = local read "HP Switcher Address"() -> (w62:i32)
                              n398 = call "HP3488A Reset(GPIB).vi"("Address"=w62, "GPIB#"=0 ("GPIB Bus")) -> ()  [unwired: 3 in, 1 out]
                            }
                          }
                        }
                        frame #1 {
                          n399 = Wait (ms)(milliseconds to wait=u32 500) -> ()  [unwired: 1 out]
                        }
                        frame #2 {
                          n400 = Greater?(x=w73, y=16) -> (0:w67:bool)
                          n401 = local read "Channel(s) (out)"() -> (w66:u16)
                          n402 = case shown="1" w66 {
                            tunnel: [w84 enum16{"Channel 1", "Channel 2", "Channel 3"}."Channel 1" ("Channel(1,2,3)") enum16{"Channel 1", "Channel 2", "Channel 3"}."Channel 2" ("Channel(1,2,3)") enum16{"Channel 1", "Channel 2", "Channel 3"}."Channel 3" ("Channel(1,2,3)")] -> w68
                            tunnel: w67 -> [w83 _ _ _]
                            frame 0, Default {
                              n403 = case shown="True" w83 {
                                tunnel: [enum16{"Channel 1", "Channel 2", "Channel 3"}."Channel 1" ("Channel(1,2,3)") enum16{"Channel 1", "Channel 2", "Channel 3"}."Channel 2" ("Channel(1,2,3)")] -> w84
                                frame False {
                                }
                                frame True {
                                }
                              }
                            }
                            frame 1 {
                            }
                            frame 2 {
                            }
                            frame 3 {
                            }
                          }
                          n404 = local read "Frequency Address"() -> (w82:i16)
                          n405 = call "HP53131 Measure Frequency2023.vi"("GPIB Bus"=0, "Number of Readings"=1, "GPIB Address"=w82, "Gate Time"=0.1, "Channel(1,2,3)"=w68) -> ("error out"=w81:errorcluster, "Frequency"=w71:dbl)  [unwired: 1 in]
                          n406 = Unbundle By Name(w81) -> ("status"=w80:bool)
                          n407 = In Range and Coerce(upper limit=5000000000.0, x=w71, lower limit=0.0) -> (coerced(x)=w74:dbl)  [unwired: 1 out]
                          n408 = case shown="True" w80 {
                            frame False {
                            }
                            frame True {
                              n409 = local read "Frequency Address"() -> (w90:i16)
                              n410 = DevClear(3:w90, 4:0 ("GPIB Bus")) -> ()  [unwired: 1 in, 2 out]
                            }
                          }
                          n411 = Not Equal?(x=w71, y=0.0) -> (x != y?=w70:bool)
                        }
                      }
                      n412 = Not(x=w46) -> (.not. x?=w47:bool)
                      n413 = local read "Halt Run"() -> (w45:bool)
                      n414 = And(x=w48, y=w47) -> (x .and. y?=w44:bool)
                      n415 = Or(x=w45, y=w44) -> (x .or. y?=w43:bool)
                    }
                  }
                }
              }
            }
            n416 = Number To Fractional String(number=w29) -> (F-format string=w30:string)  [unwired: 3 in]
          }
          frame #3 {
            n417 = local write "Functional Test Data"(w92) -> ()
            n418 = local write "Halt Run"(FALSE ("Halt Run")) -> ()
          }
        }
      }
    }
    n419 = case shown="True" w18 {
      frame False {
      }
      frame True {
        n420 = flat-sequence {
          tunnel: [w736] -> w723
          tunnel: w723 -> [w805]
          frame #0 {
            n421 = local write "Functional Test"(FALSE ("Functional Test")) -> ()
            n422 = local write "System Status"("Running Functional Test" ("System Status")) -> ()
          }
          frame #1 {
            n423 = call "Parameter Setup(Functional).vi"() -> ("Channel(s) (out)"=w726:u16, "Number of Units(out)"=w727:i32)  [unwired: 10 in]
            n424 = local write "Number of Units"(w727) -> ()
            n425 = local write "Channel(s) (out)"(w726) -> ()
          }
          frame #2 {
            n426 = Wait (ms)(milliseconds to wait=u32 500) -> ()  [unwired: 1 out]
          }
          frame #3 {
            n427 = flat-sequence {
              frame #0 {
                n428 = local read "HP Switcher Address"() -> (w729:i32)
                n429 = DevClear(3:w729, 4:0 ("GPIB Bus")) -> ()  [unwired: 1 in, 2 out]
              }
              frame #1 {
                n430 = local read "Oven Address"() -> (w731:i32)
                n431 = DevClear(3:w731, 4:0 ("GPIB Bus")) -> ()  [unwired: 1 in, 2 out]
              }
              frame #2 {
                n432 = local read "Frequency Address"() -> (w733:i16)
                n433 = DevClear(3:w733, 4:0 ("GPIB Bus")) -> ()  [unwired: 1 in, 2 out]
              }
            }
          }
          frame #4 {
            n434 = Wait (ms)(milliseconds to wait=u32 500) -> ()  [unwired: 1 out]
          }
          frame #5 {
            n435 = local read "Number of Units"() -> (w738:i32)
            n436 = for {
              N: w738 -> [_]
              shift-right: [w747] -> w736
              shift-left: "" -> [w746]
              i -> [w741]
              stop <- w739 stop-if-true
              n437 = Increment(x=w741) -> (x+1=w740:i32)
              n438 = flat-sequence {
                tunnel: w740 -> [w750]
                tunnel: [w750] -> w742
                tunnel: [w753] -> w748
                tunnel: w742 -> [w752]
                frame #0 {
                  n439 = Wait (ms)(milliseconds to wait=u32 100) -> ()  [unwired: 1 out]
                }
                frame #1 {
                  n440 = for {
                    N: 10 -> [_]
                    tunnel: w752 -> [w761]
                    tunnel: [w760] -> w753
                    stop <- w754 stop-if-true
                    n441 = flat-sequence {
                      tunnel: w761 -> [w765]
                      tunnel: [w765] -> w763
                      tunnel: [w764] -> w757
                      tunnel: [w776] -> w762
                      tunnel: w763 -> [w776]
                      tunnel: [w786] -> w760
                      tunnel: w762 -> [w785]
                      tunnel: [w782] -> w759
                      frame #0 {
                        n442 = local read "HP Switcher Address"() -> (w771:i32)
                        n443 = Bundle("GPIB Bus"=0, "HP Switcher Address"=w771) -> (w772:T1)  [unwired: 1 in]
                        n444 = call "Close HP3488A Switcher(GPIB).vi"("Device In"=w772, "reset"=FALSE, "Use Card# 5"=TRUE, "ID query"=FALSE, "error in (no error)"=errorcluster {"status"=FALSE, "code"=0, "source"=""}, "Position Number"=w765) -> ("error out"=w773:errorcluster)  [unwired: 2 in]
                        n445 = Unbundle By Name(w773) -> ("status"=w764:bool)
                        n446 = case shown="True" w764 {
                          frame False {
                          }
                          frame True {
                            n447 = local read "HP Switcher Address"() -> (w774:i32)
                            n448 = call "HP3488A Reset(GPIB).vi"("Address"=w774, "GPIB#"=0 ("GPIB Bus")) -> ()  [unwired: 3 in, 1 out]
                          }
                        }
                      }
                      frame #1 {
                        n449 = Wait (ms)(milliseconds to wait=u32 500) -> ()  [unwired: 1 out]
                      }
                      frame #2 {
                        n450 = Greater?(x=w785, y=16) -> (0:w779:bool)
                        n451 = local read "Channel(s) (out)"() -> (w778:u16)
                        n452 = case shown="0, Default" w778 {
                          tunnel: [w796 enum16{"Channel 1", "Channel 2", "Channel 3"}."Channel 1" ("Channel(1,2,3)") enum16{"Channel 1", "Channel 2", "Channel 3"}."Channel 2" ("Channel(1,2,3)") enum16{"Channel 1", "Channel 2", "Channel 3"}."Channel 3" ("Channel(1,2,3)")] -> w780
                          tunnel: w779 -> [w795 _ _ _]
                          frame 0, Default {
                            n453 = case shown="True" w795 {
                              tunnel: [enum16{"Channel 1", "Channel 2", "Channel 3"}."Channel 1" ("Channel(1,2,3)") enum16{"Channel 1", "Channel 2", "Channel 3"}."Channel 2" ("Channel(1,2,3)")] -> w796
                              frame False {
                              }
                              frame True {
                              }
                            }
                          }
                          frame 1 {
                          }
                          frame 2 {
                          }
                          frame 3 {
                          }
                        }
                        n454 = local read "Frequency Address"() -> (w794:i16)
                        n455 = call "HP53131 Measure Frequency2023.vi"("GPIB Bus"=0, "Number of Readings"=1, "GPIB Address"=w794, "Gate Time"=0.1, "Channel(1,2,3)"=w780) -> ("error out"=w793:errorcluster, "Frequency"=w783:dbl)  [unwired: 1 in]
                        n456 = Unbundle By Name(w793) -> ("status"=w792:bool)
                        n457 = In Range and Coerce(upper limit=5000000000.0, x=w783, lower limit=0.0) -> (coerced(x)=w786:dbl)  [unwired: 1 out]
                        n458 = case shown="True" w792 {
                          frame False {
                          }
                          frame True {
                            n459 = local read "Frequency Address"() -> (w802:i16)
                            n460 = DevClear(3:w802, 4:0 ("GPIB Bus")) -> ()  [unwired: 1 in, 2 out]
                          }
                        }
                        n461 = Not Equal?(x=w783, y=0.0) -> (x != y?=w782:bool)
                      }
                    }
                    n462 = Not(x=w757) -> (.not. x?=w758:bool)
                    n463 = local read "Halt Run"() -> (w756:bool)
                    n464 = And(x=w759, y=w758) -> (x .and. y?=w755:bool)
                    n465 = Or(x=w756, y=w755) -> (x .or. y?=w754:bool)
                  }
                }
              }
              n466 = Number To Fractional String(number=w748) -> (F-format string=w745:string)  [unwired: 3 in]
              n467 = Concatenate Strings(w745, "\r\n") -> (w743:string)
              n468 = local read "Halt Run"() -> (w739:bool)
              n469 = Concatenate Strings(w746, w743) -> (w747:string)
            }
          }
          frame #6 {
            n470 = local write "Halt Run"(FALSE ("Halt Run")) -> ()
            "Functional Test Data" <- w805
          }
        }
      }
    }
    n471 = local read "Exit"() -> (w15:bool)
  }
  n472 = local write "Single Func Test"(w1) -> ()
  n473 = local write "Warmup"(w1) -> ()
  n474 = local write "Halt Run"(w1) -> ()
  n475 = local write "CompRun"(w1) -> ()
  n476 = local write "Start run"(w1) -> ()
  n477 = local write "Functional Test"(w1) -> ()
  n478 = local write "Exit"(w1) -> ()
  n479 = case shown="True" w2 {
    frame False {
    }
    frame True {
      n480 = invoke class="VI" method="FP.Close"() -> ()  [unwired: 3 in, 3 out]
    }
  }
  "Chamber" <- cluster{"GPIB #":u8, "Address":u8} {"GPIB #"=0, "Address"=6} ("Chamber")
  "All Data" <- string[][][] [] ("All Data")
  "Oven Address" <- 6 ("Oven Address")
  "HP Switcher Address" <- 3 ("Bliley Switcher Address")
  "Frequency Address" <- i16 8 ("Frequency Address")
  "System" <- "BTI-BILL3" ("System")
  "Gatetime" <- "1" ("Gatetime")
